vi "Less Than.vi"(1 "comparable b":T1, 2 "comparable a":T1, 3 "connection sorter in":refnum<class "Connection Sorter By Site.lvclass">) -> (0 "less?":bool)   [LabVIEW 2020, in "MeasurementLink Session Management.lvlib" / "Connection Sorter By Site.lvclass"]
uses:
  Connection Sorter By Site.lvclass
  Session Reservation/Connection with Session.ctl
  Session Reservation/Connection.ctl
  Session Reservation/Session Reservation.lvclass
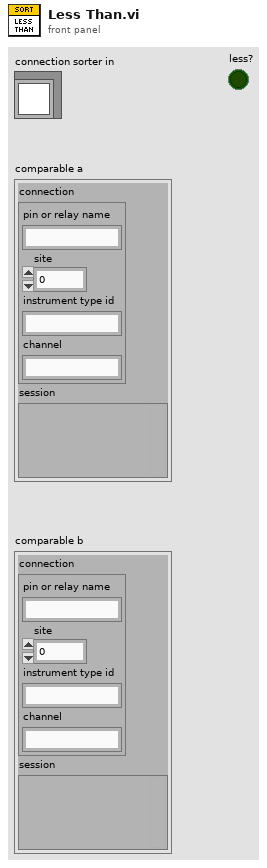
[diagram p1: front panel]
types:
  T1 = typedef "MeasurementLink Session Management.lvlib/Session Reservation.lvclass/Connection with Session.ctl" = cluster{"connection":T2, "session":variant}
  T2 = typedef "MeasurementLink Session Management.lvlib/Session Reservation.lvclass/Connection.ctl" = cluster{"pin or relay name":string, "site":i32, "instrument type id":string, "channel":string}
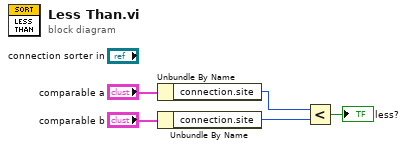
[diagram p0: block diagram]
diagram:
  n1 = Unbundle By Name("comparable a") -> ("connection.site"=w3:i32)
  n2 = Unbundle By Name("comparable b") -> ("connection.site"=w2:i32)
  n3 = Less?(x=w3, y=w2) -> (x < y?=→"less?":bool)
